vi "Write QMH Payload.vi"(8 "error in (no error)":errorcluster, 10 "Payload":variant, 11 "QMHMessagePayload in":refnum<class "QMHMessagePayload.lvclass">) -> (0 "error out":errorcluster, 3 "QMHMessagePayload out":refnum<class "QMHMessagePayload.lvclass">)   [LabVIEW 2016, in "QMHMessagePayload.lvclass"]
uses:
  QMHMessagePayload.lvclass
  QMHMessagePayload.lvclass/QMHMessagePayload.ctl
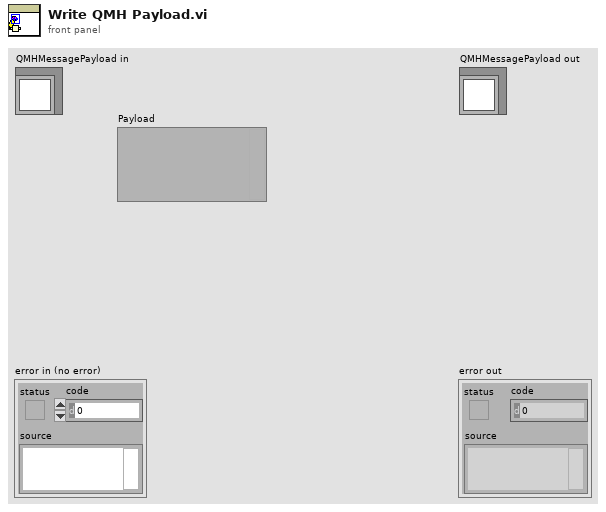
[diagram p1: front panel]
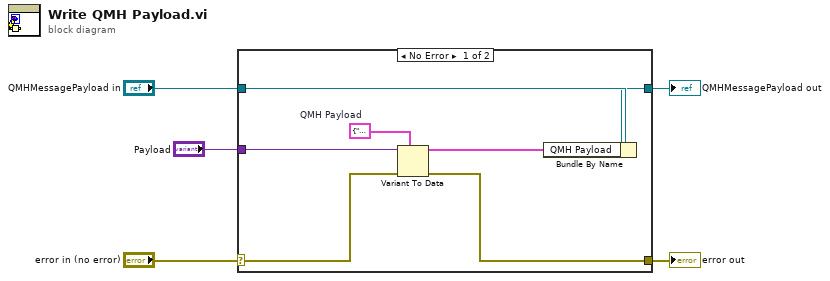
[diagram p0: block diagram]
diagram:
  n1 = case shown="No Error" "error in (no error)" {
    selector: "error in (no error)" -> [w8 w13]
    tunnel: [w7 w13] -> w4
    tunnel: [w11 w14] -> w2
    tunnel: "QMHMessagePayload in" -> [w12 w14]
    tunnel: "Payload" -> [w9 _]
    frame No Error {
      w10 = cluster{"State":enum16{""}, "Data":variant} {"State"=enum."", "Data"=variant}  # QMH Payload
      n2 = Variant To Data(error in=w8, type=w10, Variant=w9) -> (data=w6:cluster{"State":enum16{""}, "Data":variant}, error out=w7:errorcluster)
      n3 = Bundle By Name(cluster=w12, "QMH Payload"=w6) -> (w11:refnum<class "QMHMessagePayload.lvclass">)
    }
    frame Error {
    }
  }
  "error out" <- w4
  "QMHMessagePayload out" <- w2
